vi "Set DDS Trigger Source.vi"(8 "error in (no error)":errorcluster, 10 "src":u32, 11 "channel_index":u8) -> (0 "error out":errorcluster)   [LabVIEW 2021, in "vmmso.lvlib"]
doc: "DLL_API void WINAPI SetDDSTriggerSource(unsigned char channel_index, unsigned int src);"
uses:
  vmmso.lvlib
  vmmso.dll
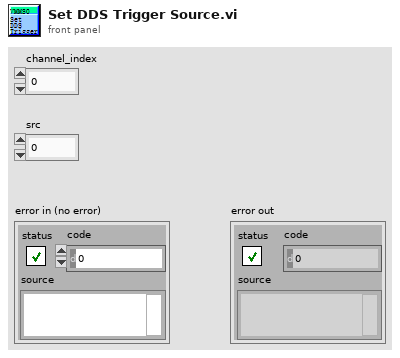
[diagram p1: front panel]
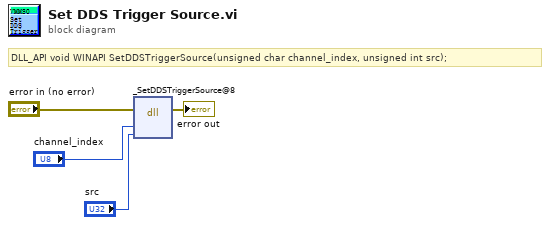
[diagram p0: block diagram]
diagram:
  # "DLL_API void WINAPI SetDDSTriggerSource(unsigned char channel_index, unsigned int src);"
  n1 = dll-call lib="O:/MSO/library/demo-Labview/vmmso/vmmso.*" fn="_SetDDSTriggerSource@8"(error in="error in (no error)", "channel_index"="channel_index", "src"="src") -> (error out=→"error out":errorcluster)  [unwired: 5 in, 1 out]
